vi "State_Machine.vi"(8 "error in (no error)":errorcluster caption="entrée d'erreur (pas d'erreur)", 11 "Delay en entrée":refnum<class "additional_information_generation_SIN.lvclass">) -> (0 "error out":errorcluster caption="sortie d'erreur", 2 "Json_String":string, 3 "Delay en sortie":refnum<class "additional_information_generation_SIN.lvclass">)   [LabVIEW 2020, in "Library Test.lvlib" / "additional_information_generation_SIN.lvclass"]
uses:
  additional_information_generation_SIN.lvclass
  Commun VI/TypeDef/Variable Printable.ctl
  JSON API/Variant JSON/Variant to JSON.vi
  JSON API/JSON Value/Get Item by name array.vi
  JSON API/JSON Value/JSON Value.lvclass
  Commun VI/Library Commun.lvlib
  JSON API/Get Polymorphic/JSON GetSet.lvlib
  JSON API/Variant JSON/Variant JSON.lvlib
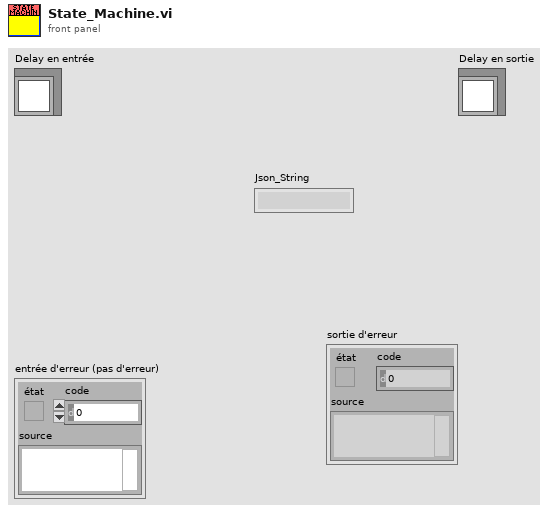
[diagram p1: front panel]
types:
  T1 = enum16{"Get Variable", "Get All Variables", "Set Variable", "Delete Variable", "Delete All Variable"}
  T2 = typedef "Variable Printable.ctl" = string
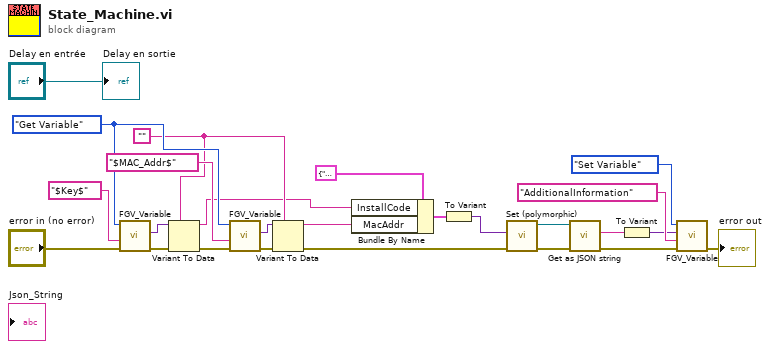
[diagram p0: block diagram]
diagram:
  w16 = ""
  w19 = T1."Get Variable" ("Function")
  n1 = call "FGV_Variable.vi"("error in (no error)"="error in (no error)", "Variable"=T2 "$Key$", "Function"=w19) -> ("error out"=w23:errorcluster, "Data Out"=w14:variant)  [unwired: 6 in, 1 out]
  n2 = Variant To Data(error in=w23, type=w16, Variant=w14) -> (data=w7:string, error out=w17:errorcluster)
  n3 = call "FGV_Variable.vi"("error in (no error)"=w17, "Variable"=T2 "$MAC_Addr$", "Function"=w19) -> ("error out"=w18:errorcluster, "Data Out"=w15:variant)  [unwired: 6 in, 1 out]
  n4 = Variant To Data(error in=w18, type=w16, Variant=w15) -> (data=w3:string, error out=w5:errorcluster)
  n5 = Bundle By Name(cluster=cluster{"MacAddr":string, "InstallCode":string} {"MacAddr"="", "InstallCode"=""}, "InstallCode"=w7, "MacAddr"=w3) -> (w6:cluster{"MacAddr":string, "InstallCode":string})
  n6 = To Variant(anything=w6) -> (Variant=w11:variant)
  n7 = call-poly "Set (polymorphic).vi"("error in (no error)"=w5, "Variant"=w11) -> ("error out"=w9:errorcluster, "JSON Value out"=w10:refnum<class "JSON Value.lvclass">)  [unwired: 8 in]
  n8 = call "Get as JSON string.vi"("error in (no error)"=w9, "JSON Value in"=w10) -> ("error out"=w4:errorcluster, "<JSON>"=w2:string)  [unwired: 8 in]
  n9 = To Variant(anything=w2) -> (Variant=w1:variant)
  n10 = call "FGV_Variable.vi"("error in (no error)"=w4, "Variable"=T2 "AdditionalInformation", "Data In"=w1, "Function"=T1."Set Variable") -> ("error out"=→"error out":errorcluster)  [unwired: 5 in, 2 out]
  "Delay en sortie" <- "Delay en entrée"
